vi "Translator.Init.vi"(8 "error in":errorcluster, 10 "Language in":string, 11 "Translation folder":path=path "D:/PL_0125_Sapphire_Automation/settings") -> (0 "error out":errorcluster, 2 "Language out":string)   [LabVIEW 2019, in "Tools.lvlib"]
uses:
  Tools.lvlib
  Translator.Global.vi
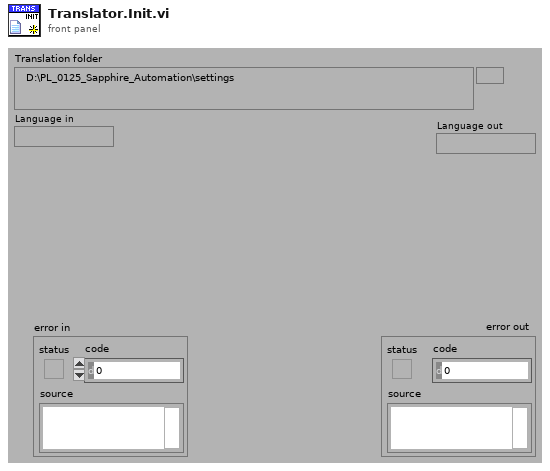
[diagram p1: front panel]
types:
  T1 = enum32{"invalid app kind", "Development System", "Run Time System", "Student Edition", "Embedded LabVIEW", "Evaluation", "Custom"}
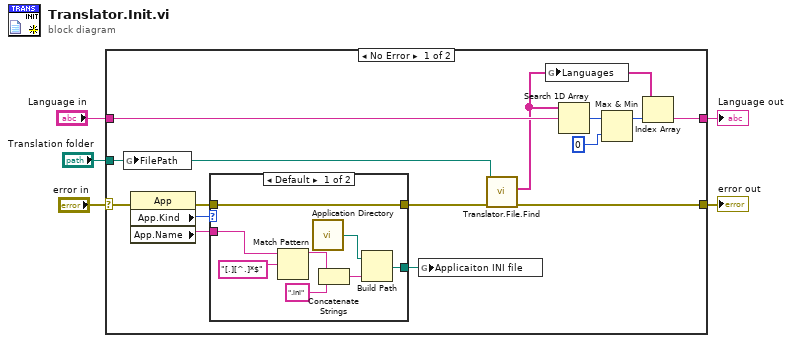
[diagram p0: block diagram]
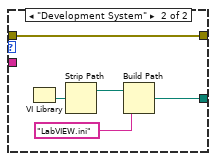
[diagram p2: hidden frame]
diagram:
  n1 = case shown="No Error" "error in" {
    selector: "error in" -> [w17 w34]
    tunnel: [w6 w34] -> w5
    tunnel: "Translation folder" -> [w7 _]
    tunnel: "Language in" -> [w11 w33]
    tunnel: [w9 w33] -> w1
    frame No Error {
      n2 = global write "Translator.Global.vi" "FilePath"(w7) -> ()
      n3 = property class="App"(error in=w17) -> (error out=w19:errorcluster, "App.Kind"=w18:T1, "App.Name"=w8:string)  [unwired: 1 in, 1 out]
      n4 = case shown="Default" w18 {
        tunnel: [w27 w32] -> w16
        tunnel: w19 -> [w27 w32]
        tunnel: [w25 w28] -> w12
        tunnel: w8 -> [w23 _]
        frame Default {
          n5 = Match Pattern(string=w23, regular expression="[.][^.]*$") -> (before substring=w22:string)  [unwired: 4 out]
          n6 = call <vilib>:"Application Directory.vi"() -> ("Application Directory"=w26:path)
          n7 = Concatenate Strings(w22, ".ini" ("string")) -> (w20:string)
          n8 = Build Path(base path=w26, name or relative path=w20) -> (appended path=w25:path)
        }
        frame "Development System" {
          n9 = VI Library() -> (path=w31:path)
          n10 = Strip Path(path=w31) -> (stripped path=w30:path)  [unwired: 1 out]
          n11 = Build Path(base path=w30, name or relative path="LabVIEW.ini") -> (appended path=w28:path)
        }
      }
      n12 = global write "Translator.Global.vi" "Applicaiton INI file"(w12) -> ()
      n13 = call "Translator.File.Find.vi"("error in"=w16, "Translation folder"=w7) -> ("error out"=w6:errorcluster, "Languages"=w10:string[])  [unwired: 8 in]
      n14 = global write "Translator.Global.vi" "Languages"(w10) -> ()
      n15 = Search 1D Array(1D array=w10, element=w11) -> (index of element=w13:i32)  [unwired: 1 in]
      n16 = Max & Min(x=w13, y=0) -> (max(x,y)=w14:i32)  [unwired: 1 out]
      n17 = Index Array(array=w10, index=w14) -> (element=w9:string)
    }
    frame Error {
    }
  }
  "error out" <- w5
  "Language out" <- w1
